vi "get TextSummary.vi"(8 "error in (no error)":errorcluster, 11 "Packet in":refnum<class "Packet.lvclass">) -> (0 "error out":errorcluster, 2 "Text Summary":string, 3 "Packet out":refnum<class "Packet.lvclass">)   [LabVIEW 2013, in "Packet.lvclass"]
doc: "Text Summary is the string that appears in the second column of the tree control. It summaries the state of the xceDataNode."
uses:
  Packet.lvclass
  xCE/xceDataNode/xceDataNode.lvclass
  xCE/xceNode/xceNode.lvclass
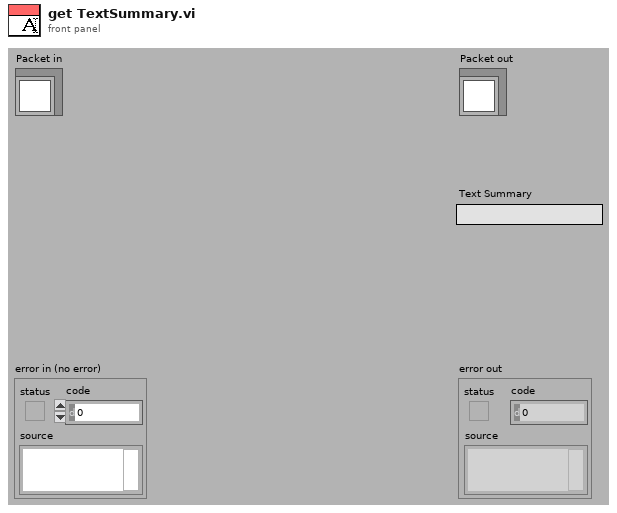
[diagram p1: front panel]
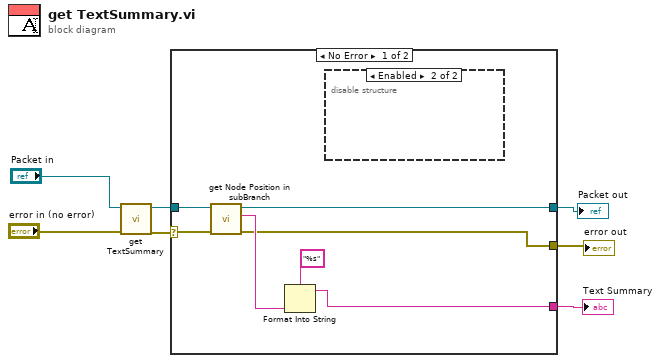
[diagram p0: block diagram]
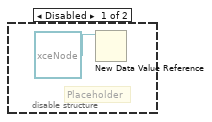
[diagram p2: hidden frame]
diagram:
  n1 = call-parent "get TextSummary.vi"("error in (no error)"="error in (no error)", "xceDataNode in"="Packet in") -> ("error out"=w4:errorcluster, "xceDataNode out"=w5:refnum<class "Packet.lvclass">)  [unwired: 7 in, 1 out]
  n2 = case shown="No Error" w4 {
    selector: w4 -> [w11 w16]
    tunnel: w5 -> [w12 w17]
    tunnel: [w8 w17] -> w3
    tunnel: [w9 w16] -> w2
    tunnel: [w13 _] -> w1
    frame No Error {
      n3 = call "get Node Position in subBranch.vi"("error in (no error)"=w11, "xceDataNode in"=w12) -> ("error out"=w9:errorcluster, "Position"=w10:string, "xceDataNode out"=w8:refnum<class "Packet.lvclass">)  [unwired: 7 in]
      n4 = Format Into String(format string="%s", w10) -> (resulting string=w13:string)  [unwired: 2 in, 1 out]
      n5 = disable-structure shown="Enabled" {
        frame Disabled {
          # "Placeholder"
          n6 = New Data Value Reference(data value=refnum<class "xceNode.lvclass"> refnum ("xceNode.lvclass")) -> ()  [unwired: 1 in, 2 out]
        }
        frame Enabled {
        }
      }
    }
    frame Error {
    }
  }
  "error out" <- w2
  "Packet out" <- w3
  "Text Summary" <- w1
